vi "2039_AccelSpike.vi"(8 "error in (no error)":errorcluster, 9 "Threshold":dbl, 10 "Delta Array":dbl[](array[numeric]), 11 "AccelerometerDevRef":T1={"DevStatus"={"status"=FALSE, "code"=0, "source"=""}, "Scaling"={"Gain (VoltsPerG)"=0.0, "Center Voltage"=0.0}, "Analog Channels"={"X-Axis"=enum."Invalid", "Y-Axis"=enum."Invalid", "Z-Axis"=enum."Invalid"}, "I2C Bus"=enum."Invalid", "SPI Bus"=enum."Invalid", "Accel Range"=0, "ADXL Axes"={"X-Axis"=FALSE, "Y-Axis"=FALSE, "Z-Axis"=FALSE}, "Handle"=0, "Device Address"=0, "Accel Type"=enum."Analog"} {"Device Address" format="%.0x"; "Accel Range" items=["+/- 2 g", "+/- 4 g", "+/- 8 g", "+/- 16 g"]}) -> (0 "error out":errorcluster, 2 "Event Registration Refnum":refnum<event-registration>)   [LabVIEW 2015]
uses:
  <vilib>/Rock Robotics/WPI/Accelerometer/WPI_AccelerometerDevRef.ctl
  <vilib>/Rock Robotics/WPI/Accelerometer/WPI_AccelerometerScaling.ctl
  <vilib>/Rock Robotics/WPI/Accelerometer/WPI_AccelerometerAnalogChannels.ctl
  <vilib>/Rock Robotics/SystemInterfaces/AI/FPGA_AIChannel.ctl
  <vilib>/Rock Robotics/SystemInterfaces/i2clib/i2c_bus.ctl
  <vilib>/Rock Robotics/SystemInterfaces/spilib/spi_bus.ctl
  <vilib>/Rock Robotics/WPI/Accelerometer/ADXL345 Range.ctl
  <vilib>/Rock Robotics/WPI/Accelerometer/WPI_AccelerometerADXL345 Axes.ctl
panel:
  # "ADXL"
  # "Analog"
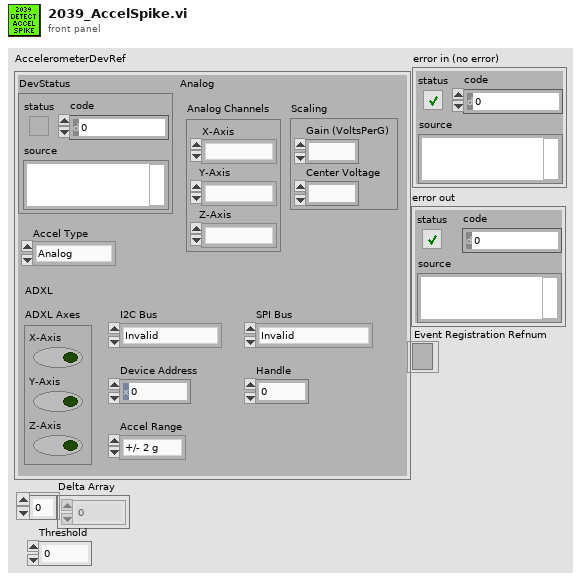
[diagram p1: front panel]
types:
  T1 = typedef "WPI_AccelerometerDevRef.ctl" = cluster{"DevStatus":errorcluster, "Scaling":T2, "Analog Channels":T3, "I2C Bus":T5, "SPI Bus":T6, "Accel Range":T7, "ADXL Axes":T8, "Handle":i32, "Device Address":u8, "Accel Type":enum16{"Analog", "ADXL345 I2C", "ADXL345 SPI", "Internal", "ADXL362 SPI"}}
  T2 = typedef "WPI_AccelerometerScaling.ctl" = cluster{"Gain (VoltsPerG)":dbl, "Center Voltage":dbl}
  T3 = typedef "WPI_AccelerometerAnalogChannels.ctl" = cluster{"X-Axis":T4, "Y-Axis":T4, "Z-Axis":T4}
  T4 = typedef "FPGA_AIChannel.ctl" = enum8{"AI 0", "AI 1", "AI 2", "AI 3", "AI MXP 0", "AI MXP 1", "AI MXP 2", "AI MXP 3", "Invalid"}
  T5 = typedef "i2c_bus.ctl" = enum16{"I2C On-Board", "I2C MXP", "Invalid"}
  T6 = typedef "spi_bus.ctl" = enum16{"SPI On-Board, CS0", "SPI On-Board, CS1", "SPI On-Board, CS2", "SPI On-Board, CS3", "SPI MXP", "Invalid"}
  T7 = typedef "ADXL345 Range.ctl" = u8
  T8 = typedef "WPI_AccelerometerADXL345 Axes.ctl" = cluster{"X-Axis":bool, "Y-Axis":bool, "Z-Axis":bool}
  T9 = cluster{"X-Axis":dbl, "Y-Axis":dbl, "Z-Axis":dbl}
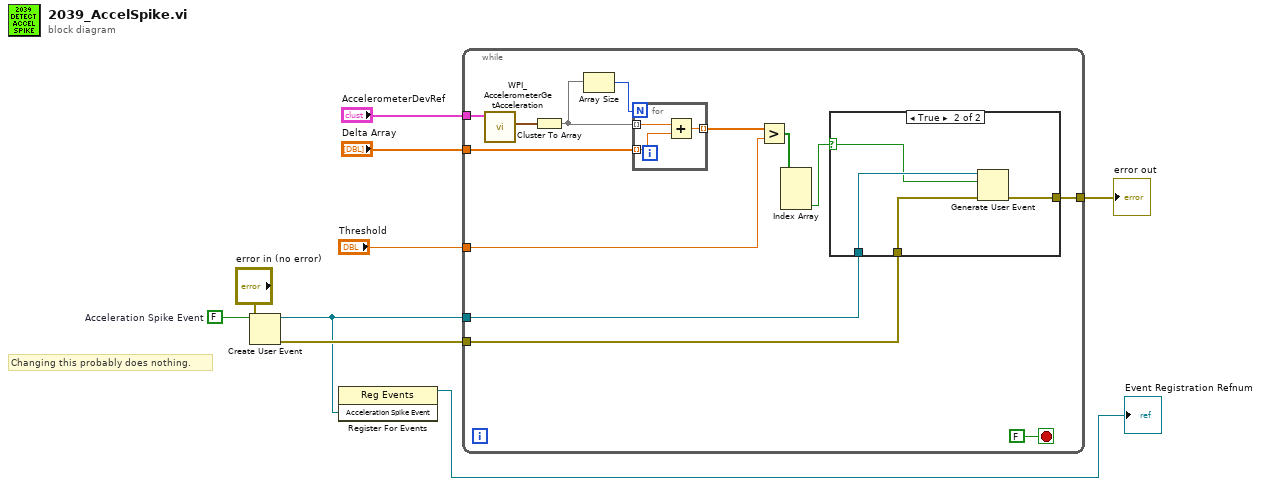
[diagram p0: block diagram]
diagram:
  w6 = FALSE  # Acceleration Spike Event
  # "Changing this probably does nothing."
  n1 = Create User Event(user event datatype=w6, error in="error in (no error)") -> (user event=w2:refnum<user-event>, error out=w5:errorcluster)
  n2 = register-events(w2) -> (reference out=→"Event Registration Refnum":refnum<event-registration>)  [unwired: 2 in, 1 out]
  n3 = while {
    tunnel: "AccelerometerDevRef" -> [w20]
    tunnel: "Delta Array" -> [w18]
    tunnel: "Threshold" -> [w16]
    tunnel: w2 -> [w13]
    tunnel: w5 -> [w12]
    tunnel: [w11] -> w3
    stop <- FALSE stop-if-true
    n4 = call <vilib>:"WPI_AccelerometerGetAcceleration.vi"("AccelerometerDevRef"=w20) -> ("Accelerations"=w21:T9)  [unwired: 8 in, 2 out]
    n5 = Cluster To Array(cluster=w21) -> (array=w19:dbl[])
    n6 = Array Size(array=w19) -> (size(s)=w22:i32)
    n7 = for {
      N: w22 -> [_]
      tunnel: w19 -> [w30] mode=indexing
      tunnel: w18 -> [w29] mode=indexing
      tunnel: [w28] -> w17 mode=indexing
      n8 = Add(x=w30, y=w29) -> (x+y=w28:dbl)
    }
    n9 = Greater?(x=w17, y=w16) -> (0:w15:bool[])
    n10 = Index Array(array=w15) -> (element #3=w14:bool)  [unwired: 3 in, 2 out]
    n11 = case shown="True" w14 {
      selector: w14 -> [_ w26]
      tunnel: w13 -> [_ w27]
      tunnel: w12 -> [w23 w25]
      tunnel: [w23 w24] -> w11
      frame False {
      }
      frame True {
        n12 = Generate User Event(user event=w27, event data cluster=w26, error in=w25) -> (error out=w24:errorcluster)  [unwired: 1 in, 1 out]
      }
    }
  }
  "error out" <- w3
